vi "Live window-Image display mapping.vi"(8 "error in (no error)":errorcluster, 9 "Intensity sliders":cluster{i16, i16}, 11 "Which image display?":T1) -> (0 "error out":errorcluster)   [LabVIEW 2013]
uses:
  Typedefs/Left-Right enum.ctl
  Globals/gl_Windows Ctrl refs.vi
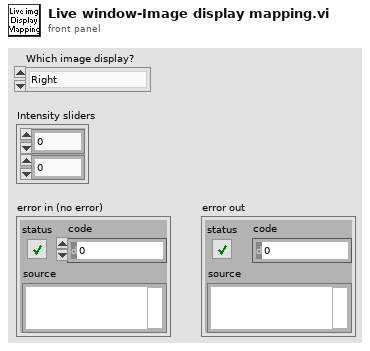
[diagram p1: front panel]
types:
  T1 = typedef "Left-Right enum.ctl" = enum16{"Right", "Left"}
  T2 = typedef "Image display ref.ctl" = refnum<vi>
  T3 = typedef "Live window-ctrl refs.ctl" = cluster{"This VI":refnum<vi>, "Pane":refnum<vi>, "Snapshot":refnum<vi>, "Left Image Palette":refnum<vi>, "Right Image Palette":refnum<vi>, "Left Channel":refnum<vi>, "Right Channel":refnum<vi>, "Left image intensity":refnum<vi>, "Right image intensity":refnum<vi>, "Left Image Display":T2, "Right Image Display":T2, "Refresh rate ind (Hz)":refnum<vi>, "Acq rate ind (Hz)":refnum<vi>, "Stop (ind)":refnum<vi>}
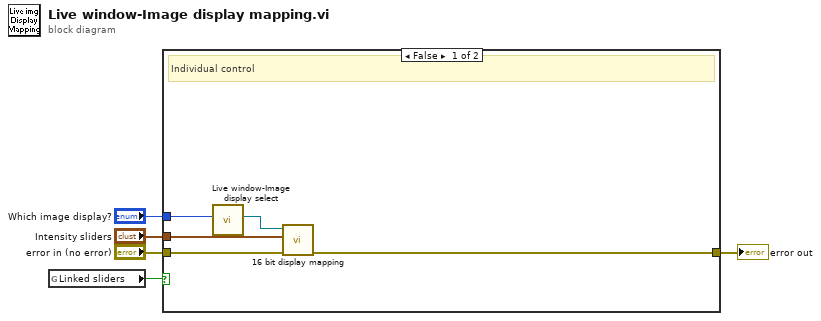
[diagram p0: block diagram]
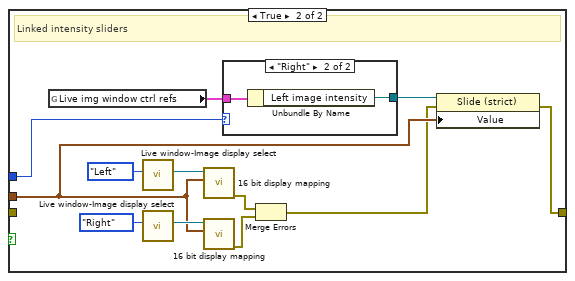
[diagram p2: hidden frame]
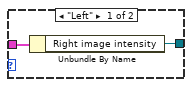
[diagram p3: hidden frame]
diagram:
  n1 = global read "gl_Windows Ctrl refs.vi" "Linked sliders"() -> (w1:bool)
  n2 = case shown="False" w1 {
    tunnel: [w10 w11] -> w5
    tunnel: "error in (no error)" -> [w9 _]
    tunnel: "Intensity sliders" -> [w8 w13]
    tunnel: "Which image display?" -> [w6 w15]
    frame False {
      # "Individual control"
      n3 = call "Live window-Image display select.vi"("Which image display?"=w6) -> ("Image display ref"=w7:T2)  [unwired: 10 in]
      n4 = call "16 bit display mapping.vi"("error in (no error)"=w9, "16 bit display mapping"=w8, "Image Display"=w7) -> ("error out"=w10:errorcluster)  [unwired: 7 in, 1 out]
    }
    frame True {
      # "Linked intensity sliders"
      n5 = global read "gl_Windows Ctrl refs.vi" "Live img window ctrl refs"() -> (w16:T3)
      n6 = call "Live window-Image display select.vi"("Which image display?"=Left-Right_enum."Left") -> ("Image display ref"=w20:T2)  [unwired: 10 in]
      n7 = call "Live window-Image display select.vi"("Which image display?"=Left-Right_enum."Right") -> ("Image display ref"=w19:T2)  [unwired: 10 in]
      n8 = call "16 bit display mapping.vi"("16 bit display mapping"=w13, "Image Display"=w20) -> ("error out"=w18:errorcluster)  [unwired: 8 in, 1 out]
      n9 = call "16 bit display mapping.vi"("16 bit display mapping"=w13, "Image Display"=w19) -> ("error out"=w17:errorcluster)  [unwired: 8 in, 1 out]
      n10 = case shown="\"Right\"" w15 {
        tunnel: w16 -> [w24 w26]
        tunnel: [w23 w25] -> w14
        frame "Left" {
          n11 = Unbundle By Name(w24) -> ("Right image intensity"=w23:refnum<vi>)
        }
        frame "Right" {
          n12 = Unbundle By Name(w26) -> ("Left image intensity"=w25:refnum<vi>)
        }
      }
      n13 = Merge Errors(w18, w17) -> (w12:errorcluster)
      n14 = property class="Slide (strict)"(reference=w14, error in=w12, "Value"=w13) -> (error out=w11:errorcluster)  [unwired: 1 out]
    }
  }
  "error out" <- w5
